vi "Auto save image.vi"(11 "Run?":bool) -> (3 "Done":bool)   [LabVIEW 2013]
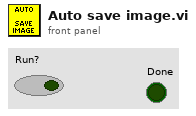
[diagram p1: front panel]
types:
  T1 = typedef "Image Type" = u32
  T2 = typedef "WPI_CameraDevRef.ctl" = cluster{"Camera Address":string, "CameraStatus":errorcluster, "Acquire Image Notifier":refnum<notifier>}
  T3 = typedef "IMAQ Image.ctl" = refnum<image>
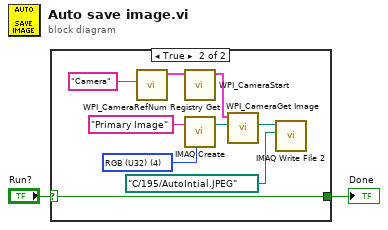
[diagram p0: block diagram]
diagram:
  n1 = case shown="True" "Run?" {
    selector: "Run?" -> [w3 w6]
    tunnel: [w3 w6] -> w1
    frame False {
    }
    frame True {
      w12 = T1 4 items=["Grayscale (U8)", "Grayscale (I16)", "Grayscale (SGL)", "Complex (CSG)", "RGB (U32)", "HSL (U32)", "RGB (U64)"] ("Image Type")
      n2 = call <vilib>:"WPI_CameraRefNum Registry Get.vi"("refnum name"="Camera") -> ("CameraDevRef"=w5:T2)  [unwired: 9 in, 1 out]
      n3 = call <vilib>:"WPI_CameraStart.vi"("CameraDevRef"=w5) -> ("CameraDevRef Out"=w9:T2)  [unwired: 9 in, 1 out]
      n4 = call "IMAQ Create"("Image Name"="Primary Image", "Image Type"=w12) -> ("New Image"=w10:T3)  [unwired: 2 in, 2 out]
      n5 = call <vilib>:"WPI_CameraGet Image.vi"("Image"=w10, "CameraDevRef"=w9) -> ("Image Out"=w8:T3)  [unwired: 1 in, 8 out]
      n6 = call-poly "IMAQ Write File 2"("File Path"=path "C:/195/AutoIntial.JPEG", "Image"=w8) -> ()  [unwired: 8 in, 2 out]
    }
  }
  "Done" <- w1
